vi "test_configuration.vi"   [LabVIEW 2019, in "Inst.TC.lvclass"]
uses:
  Inst.TC.lvclass
  Inst.TC.lvclass/Inst.TC.ctl
  FP-TC-Shared/FP-TC-Shared.lvclass
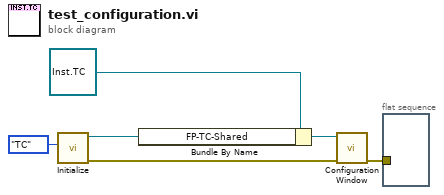
[diagram p0: block diagram]
diagram:
  n1 = call "Initialize.vi"("Application"=enum16{"TC", "FP"}."TC") -> ("error out"=w1:errorcluster, "FP-TC-Shared out"=w4:refnum<class "FP-TC-Shared.lvclass">)  [unwired: 9 in]
  n2 = Bundle By Name(cluster=refnum<class "Inst.TC.lvclass"> refnum ("Inst.TC.lvclass"), "FP-TC-Shared"=w4) -> (w3:refnum<class "Inst.TC.lvclass">)
  n3 = call-dynamic "Configuration Window.vi"("error in (no error)"=w1, "Inst.TC"=w3) -> ("error out"=w2:errorcluster)  [unwired: 8 in, 1 out]
  n4 = flat-sequence {
    tunnel: w2 -> [_]
    frame #0 {
    }
  }
